vi "配置文件write.vi"(7 "updateconfiguration":cluster{"IP地址":string, "端口号":i32, "软件版本":string}={"IP地址"="27.154.58.30", "端口号"=10050, "软件版本"=""}, 8 "error in (no error)":errorcluster caption="错误输入（无错误）", 9 "configuration file path":path caption="配置文件的路径", 10 "键数组":string[](array[string]), 11 "段":string="应用程序交互") -> (0 "error out":errorcluster caption="错误输出")   [LabVIEW 2016, in "自动更新.lvlib"]
uses:
  <vilib>/Utility/config.llb/Write Key (I32).vi
  <vilib>/Utility/config.llb/Write Key (String).vi
  <vilib>/Utility/config.llb/NI_LVConfig.lvlib
  <vilib>/Utility/Data Type/NI_Data Type.lvlib
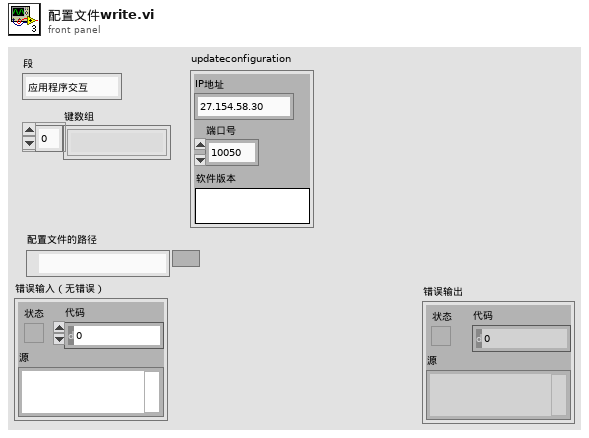
[diagram p1: front panel]
types:
  T1 = typedef "NI_LVConfig.lvlib/Config Data RefNum.ctl" = refnum<k1>
  T2 = typedef "NI_Data Type.lvlib/Data Type.ctl" = enum8{"Invalid Type", "Void", "I8", "I16", "I32", "I64", "U8", "U16", "U32", "U64", "Single Float", "Double Float", "Extended Float", "Single Complex", "Double Complex", "Extended Complex", "Enum U8", "Enum U16", "Enum U32", "Enum U64", "Single Float With Unit", "Double Float With Unit", "Extended Float With Unit", "Single Complex with Unit", "Double Complex with Unit", "Extended Complex with Unit", "Boolean", "String", "Path", "Picture", "Tag", "Array", "Cluster", "Variant", "LV Variant", "Waveform", "Timestamp", "Digital Waveform", "Digital Data", "ExpressData", "Refnum", "External Data", "VI", "Poly VI", "LabVIEW Class Instance", "Fixed Point"}
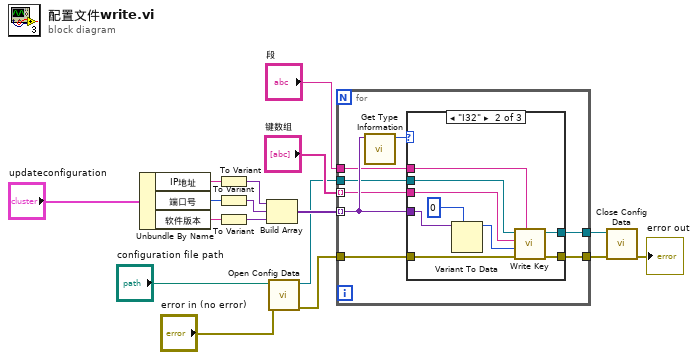
[diagram p0: block diagram]
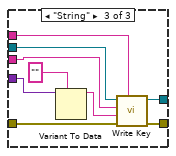
[diagram p3: hidden frame]
diagram:
  n1 = Unbundle By Name("updateconfiguration") -> ("IP地址"=w14:string, "端口号"=w13:i32, "软件版本"=w12:string)
  n2 = To Variant(anything=w14) -> (Variant=w11:variant)
  n3 = To Variant(anything=w13) -> (Variant=w9:variant)
  n4 = To Variant(anything=w12) -> (Variant=w10:variant)
  n5 = Build Array(w11, w9, w10) -> (w8:variant[])
  n6 = call <vilib>:"Open Config Data.vi"("error in (no error)"="error in (no error)", "configuration file path"="configuration file path") -> ("error out"=w6:errorcluster, "refnum"=w7:T1)  [unwired: 7 in, 1 out]
  n7 = for {
    tunnel: "键数组" -> [w20] mode=indexing
    tunnel: w8 -> [w24] mode=indexing
    tunnel: w7 -> [w23]
    tunnel: w6 -> [w22]
    tunnel: "段" -> [w21]
    tunnel: [w19] -> w4
    tunnel: [w18] -> w3
    n8 = call <vilib>:"Get Type Information.vi"("Variant"=w24) -> ("Type"=w25:T2)  [unwired: 6 in, 4 out]
    n9 = case shown="\"I32\"" w25 {
      tunnel: [w27 w34 w43] -> w19
      tunnel: [w26 w33 w42] -> w18
      tunnel: w24 -> [_ w28 w41]
      tunnel: w23 -> [w27 w32 w40]
      tunnel: w22 -> [w26 w31 w39]
      tunnel: w21 -> [_ w30 w38]
      tunnel: w20 -> [_ w29 w37]
      frame "Invalid Type", Default {
      }
      frame "I32" {
        n10 = Variant To Data(type=0, Variant=w28) -> (data=w35:i32)  [unwired: 1 in, 1 out]
        n11 = call-poly <vilib>:"Write Key.vi"("section"=w30, "error in (no error)"=w31, "value"=w35, "key"=w29, "refnum"=w32) -> ("error out"=w33:errorcluster, "refnum out"=w34:T1)  [unwired: 4 in, 1 out]
      }
      frame "String" {
        n12 = Variant To Data(type="", Variant=w41) -> (data=w44:string)  [unwired: 1 in, 1 out]
        n13 = call-poly <vilib>:"Write Key.vi"("section"=w38, "error in (no error)"=w39, "value"=w44, "key"=w37, "refnum"=w40) -> ("error out"=w42:errorcluster, "refnum out"=w43:T1)  [unwired: 4 in, 1 out]
      }
    }
  }
  n14 = call <vilib>:"Close Config Data.vi"("error in (no error)"=w3, "refnum"=w4) -> ("error out"=→"error out":errorcluster)  [unwired: 8 in, 1 out]
